vi "XIPIN_AXI_1G_2.5G_Ethernet_Subsystem_7_0.vi"   [LabVIEW 2017]
doc: "AXI 1G/2.5G Ethernet Subsystem implements a Tri-mode (10/100/1000 Mb/s) Ethernet MAC. This core supports the use of MII, GMII, SGMII, RGMII, and 1000BaseX Interfaces to connect MAC to a PHY chip. It also provides on-chip PHY in case of SGMII and 1000BaseX modes. The MDIO interface is used to access PHY Management registers. This core optionally enables 'TCP/UDP full checksum offload', 'VLAN stripping, tagging, translation' and 'Extended filtering for multicast frames' features. The AXI Ethernet core optionally supports Ethernet Audio Video Bridging (AVB) functions. The core also provide optional IEEE1588-2008 1-step and 2-step hardware time-stamping. This core provides a control interface to internal registers using AXI4-Lite interface. The transmit and receive data interfaces use AXI4-Stream interface. This core optionally supports 2.5G Ethernet.\n------------------------------------\n<b>Need License</b> : Yes\n<b>Interface</b> : AXI4 AXI4-Stream"
uses:
  <vilib>/rvi/XilinxIP/XIPIN_XNode/niFpgaXIPIN.xnode
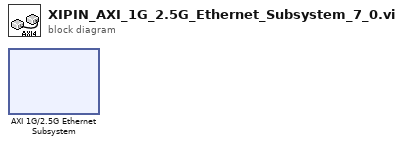
[diagram p0: block diagram]
diagram:
  n1 = xnode ("AXI 1G/2.5G Ethernet Subsystem")() -> ()
